vi "Measurement.vi"(8 "error in (no error)":errorcluster, 9 "Grandeza":string, 10 "Multiplicador":dbl, 11 "TY720 in":refnum<class "TY720.lvclass">) -> (0 "error out":errorcluster, 2 "Measurement":dbl, 3 "TY720 out":refnum<class "TY720.lvclass">)   [LabVIEW 2015, in "TY720.lvclass"]
doc: "VI used to measure Value using the multimeter"
uses:
  TY720.lvclass
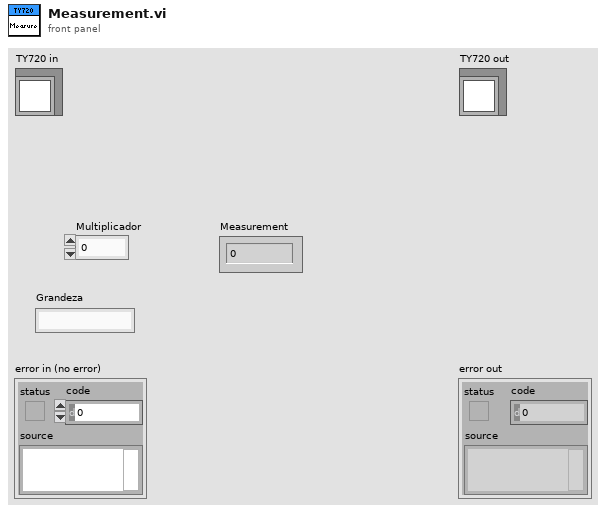
[diagram p1: front panel]
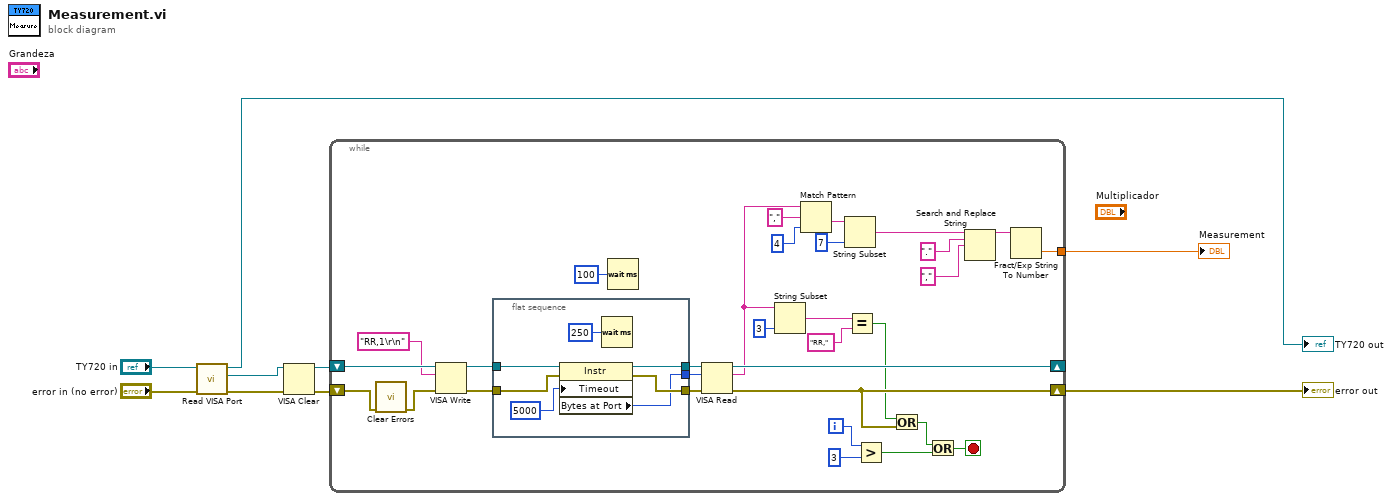
[diagram p0: block diagram]
diagram:
  n1 = call-dynamic "Read VISA Port.vi"("error in (no error)"="error in (no error)", "Device in"="TY720 in") -> ("error out"=w7:errorcluster, "VISA Port"=w1:refnum<visa-resource-name>, "Device out"=→"TY720 out":refnum<class "TY720.lvclass">)  [unwired: 7 in]
  n2 = VISA Clear(VISA resource name=w1, error in (no error)=w7) -> (VISA resource name out=w8:refnum<visa-resource-name>, error out=w9:errorcluster)
  n3 = while {
    shift-right: [w25] -> w6
    shift-left: w9 -> [w31]
    shift-right: [w39] -> _
    shift-left: w8 -> [w40]
    tunnel: [w14] -> w2
    i -> [w33]
    stop <- w26 stop-if-true
    n4 = call <vilib>:"Clear Errors.vi"("error in (no error)"=w31) -> ("error out"=w30:errorcluster)  [unwired: 5 in, 1 out]
    n5 = VISA Write(VISA resource name=w40, write buffer="RR,1\r\n", error in (no error)=w30) -> (VISA resource name out=w37:refnum<visa-resource-name>, error out=w35:errorcluster)  [unwired: 1 out]
    n6 = flat-sequence {
      tunnel: w37 -> [w47]
      tunnel: [w45] -> w36
      tunnel: w35 -> [w44]
      tunnel: [w43] -> w34
      tunnel: [w42] -> w23
      frame #0 {
        n7 = property class="Instr"(reference=w47, error in=w44, "Timeout"=u32 5000 ("General Settings:Timeout Value")) -> (reference out=w45:refnum<visa-resource-name>, error out=w43:errorcluster, "Bytes at Port"=w42:u32)
        n8 = Wait (ms)(milliseconds to wait=u32 250) -> ()  [unwired: 1 out]
      }
    }
    n9 = Wait (ms)(milliseconds to wait=u32 100) -> ()  [unwired: 1 out]
    n10 = VISA Read(VISA resource name=w36, byte count=w23, error in (no error)=w34) -> (VISA resource name out=w39:refnum<visa-resource-name>, read buffer=w19:string, error out=w25:errorcluster)  [unwired: 1 out]
    n11 = String Subset(string=w19, length (rest)=3 ("length (rest)")) -> (substring=w20:string)  [unwired: 1 in]
    n12 = Match Pattern(string=w19, regular expression=",", offset (0)=4) -> (after substring=w15:string)  [unwired: 3 out]
    n13 = String Subset(string=w15, length (rest)=7 ("offset (0)")) -> (substring=w12:string)  [unwired: 1 in]
    n14 = Equal?(x=w20, y="RR,") -> (x = y?=w22:bool)
    n15 = Greater?(x=w33, y=3) -> (0:w27:bool)
    n16 = Or(x=w22, y=w25) -> (x .or. y?=w24:bool)
    n17 = Or(x=w24, y=w27) -> (x .or. y?=w26:bool)
    n18 = Search and Replace String(input string=w12, search string=".", replace string="," ("search string")) -> (result string=w10:string)  [unwired: 5 in, 3 out]
    n19 = Fract/Exp String To Number(string=w10) -> (number=w14:dbl)  [unwired: 3 in, 1 out]
  }
  "error out" <- w6
  "Measurement" <- w2
